vi "Client Pool FGV.vi"(8 "error in (no error)":errorcluster, 11 "Client":T1) -> (0 "error out":errorcluster, 3 "grpc client id":T2)   [LabVIEW 2020, in "MeasurementLink Measurement Server.lvlib" / "ClientPool.lvclass"]
uses:
  ClientPool.lvclass
  ClientPool.lvclass/ClientPool.ctl
  <vilib>/gRPC/LabVIEW gRPC Library/Shared/grpcId.ctl
  <vilib>/gRPC/LabVIEW gRPC Library/grpc-lvsupport-release.lvlib
  FGV Action.ctl
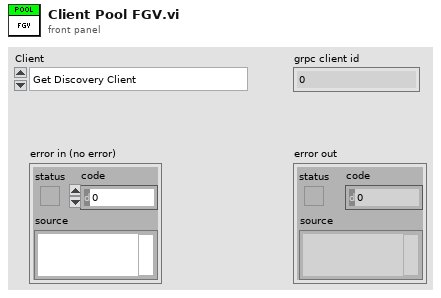
[diagram p1: front panel]
types:
  T1 = typedef "MeasurementLink Measurement Server.lvlib/ClientPool.lvclass/FGV Action.ctl" = enum16{"Get Discovery Client", "Get Session Client", "Get Pinmap Client"}
  T2 = typedef "grpc-lvsupport-release.lvlib/grpcId.ctl" = u64
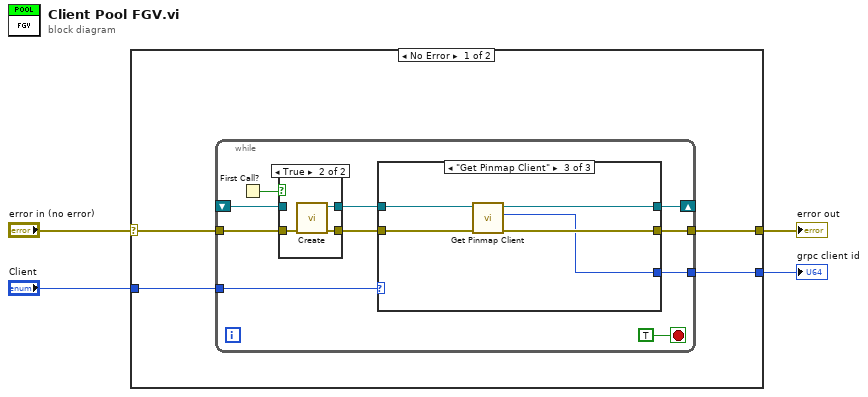
[diagram p0: block diagram]
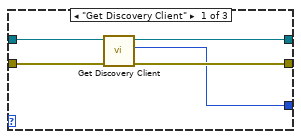
[diagram p3: hidden frame]
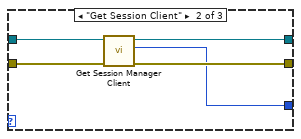
[diagram p4: hidden frame]
diagram:
  n1 = case shown="No Error" "error in (no error)" {
    selector: "error in (no error)" -> [w7 w39]
    tunnel: [w8 w39] -> w3
    tunnel: [w6 _] -> w2
    tunnel: "Client" -> [w5 _]
    frame No Error {
      n2 = while {
        tunnel: [w11] -> w8
        shift-right: [w13] -> _
        shift-left: _ -> [w15]
        tunnel: w7 -> [w17]
        tunnel: [w10] -> w6
        tunnel: w5 -> [w9]
        stop <- TRUE stop-if-true
        n3 = First Call?() -> (First Call?: T/F=w16:bool)
        n4 = case shown="True" w16 {
          tunnel: w17 -> [w20 w23]
          tunnel: [w20 w22] -> w12
          tunnel: [w19 w21] -> w14
          tunnel: w15 -> [w19 _]
          frame False {
          }
          frame True {
            n5 = call "Create.vi"("error in (no error)"=w23) -> ("error out"=w22:errorcluster, "ClientPool out"=w21:refnum<class "ClientPool.lvclass">)  [unwired: 9 in]
          }
        }
        n6 = case shown="\"Get Pinmap Client\"" w9 {
          tunnel: w14 -> [w27 w33 w38]
          tunnel: [w26 w32 w37] -> w13
          tunnel: w12 -> [w28 w31 w36]
          tunnel: [w25 w30 w35] -> w11
          tunnel: [w24 w29 w34] -> w10
          frame "Get Discovery Client" {
            n7 = call "Get Discovery Client.vi"("error in (no error)"=w28, "ClientPool in"=w27) -> ("error out"=w25:errorcluster, "Discovery grpc id"=w24:T2, "ClientPool out"=w26:refnum<class "ClientPool.lvclass">)  [unwired: 7 in]
          }
          frame "Get Session Client" {
            n8 = call "Get Session Manager Client.vi"("error in (no error)"=w31, "ClientPool in"=w33) -> ("error out"=w30:errorcluster, "Session manger grpc id"=w29:T2, "ClientPool out"=w32:refnum<class "ClientPool.lvclass">)  [unwired: 7 in]
          }
          frame "Get Pinmap Client" {
            n9 = call "Get Pinmap Client.vi"("error in (no error)"=w36, "ClientPool in"=w38) -> ("error out"=w35:errorcluster, "Pinmap grpc id"=w34:T2, "ClientPool out"=w37:refnum<class "ClientPool.lvclass">)  [unwired: 7 in]
          }
        }
      }
    }
    frame Error {
    }
  }
  "error out" <- w3
  "grpc client id" <- w2
